vi "ParallelForLoopDialogHelper.vi"(10 "Debugging Enabled In":bool, 11 "Parallelism Enabled In":bool) -> (2 "Disable radio buttons and num instances?":T1(ring), 3 "Disable debugging enabled checkbox?":T1(ring))   [LabVIEW 2016]
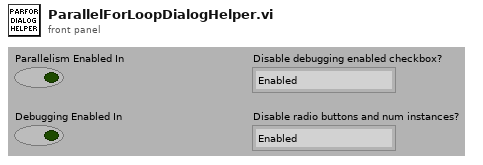
[diagram p1: front panel]
types:
  T1 = enum8{"Enabled", "Disabled", "Disabled and Grayed Out"}
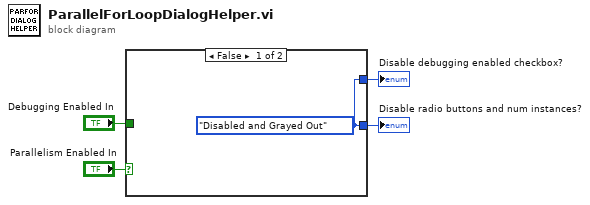
[diagram p0: block diagram]
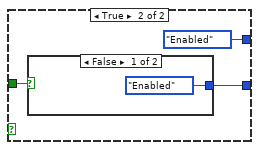
[diagram p2: hidden frame]
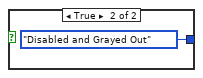
[diagram p3: hidden frame]
diagram:
  n1 = case shown="False" "Parallelism Enabled In" {
    tunnel: [w5 T1."Enabled" ("Disabled")] -> w2
    tunnel: [w5 w7] -> w3
    tunnel: "Debugging Enabled In" -> [_ w6]
    frame False {
      w5 = T1."Disabled and Grayed Out" ("Disabled")
    }
    frame True {
      n2 = case shown="False" w6 {
        tunnel: [T1."Enabled" ("Disabled") T1."Disabled and Grayed Out" ("Disabled")] -> w7
        frame False {
        }
        frame True {
        }
      }
    }
  }
  "Disable radio buttons and num instances?" <- w3
  "Disable debugging enabled checkbox?" <- w2
